vi "题目1.vi"() -> ()   [LabVIEW 2017]
panel:
  out "?":bool
  out "倒计时":string
  in  "停止":bool
  in  "开始计时":bool
  in  "定时时间选择":enum16{"90秒", "6秒", "10秒", "20秒"}(ring)
  # "倒 计 时 器"
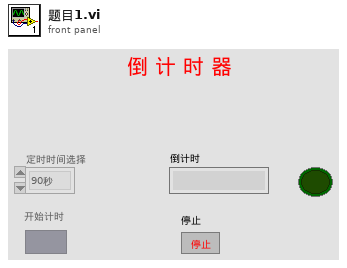
[diagram p1: front panel]
types:
  T1 = enum8{"Enabled", "Disabled", "Disabled and Grayed Out"}
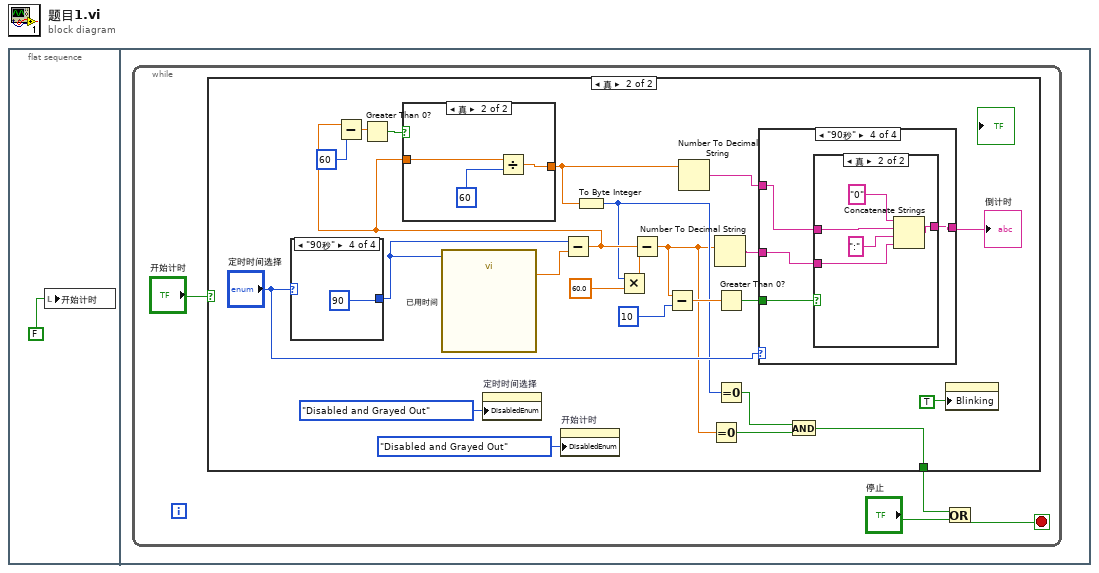
[diagram p0: block diagram]
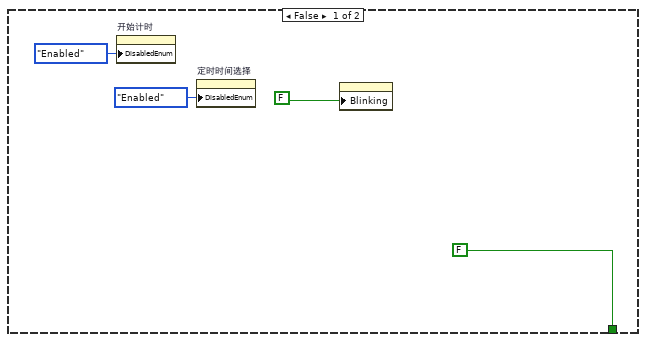
[diagram p2: hidden frame]
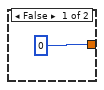
[diagram p3: hidden frame]
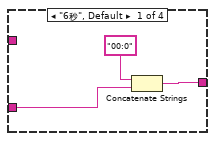
[diagram p4: hidden frame]
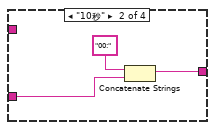
[diagram p5: hidden frame]
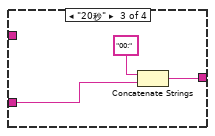
[diagram p6: hidden frame]
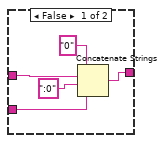
[diagram p7: hidden frame]
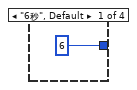
[diagram p8: hidden frame]
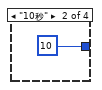
[diagram p9: hidden frame]
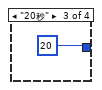
[diagram p10: hidden frame]
diagram:
  n1 = flat-sequence {
    frame #0 {
      n2 = local write "开始计时"(FALSE ("布尔")) -> ()
    }
    frame #1 {
      n3 = while {
        stop <- w2 stop-if-true
        n4 = case shown="真" "开始计时" {
          tunnel: [FALSE w12] -> w4
          frame False {
            n5 = property on="开始计时" class="Bool (严格)"("DisabledEnum"=T1."Enabled" ("禁用")) -> ()  [unwired: 2 in, 2 out]
            n6 = property on="定时时间选择" class="Enum (严格)"("DisabledEnum"=T1."Enabled" ("禁用")) -> ()  [unwired: 2 in, 2 out]
            n7 = property class="Bool (严格)"("Blinking"=FALSE ("闪烁")) -> ()  [unwired: 2 in, 2 out]
          }
          frame True {
            n8 = case shown="\"90秒\"" "定时时间选择" {
              tunnel: [6 10 20 90] -> w27
              frame "6秒", Default {
              }
              frame "10秒" {
              }
              frame "20秒" {
              }
              frame "90秒" {
              }
            }
            n9 = call "已用时间"("Time Target (s)"=w27) -> ("Elapsed Time (s)"=w25:dbl)  [unwired: 11 in, 7 out]
            n10 = property on="定时时间选择" class="Enum (严格)"("DisabledEnum"=T1."Disabled and Grayed Out" ("禁用")) -> ()  [unwired: 2 in, 2 out]
            n11 = property on="开始计时" class="Bool (严格)"("DisabledEnum"=T1."Disabled and Grayed Out" ("禁用")) -> ()  [unwired: 2 in, 2 out]
            n12 = Subtract(x=w27, y=w25) -> (x-y=w18:dbl)
            n13 = Subtract(x=w18, y=60) -> (x-y=w29:dbl)
            n14 = Greater Than 0?(x=w29) -> (x > 0?=w28:bool)
            n15 = case shown="真" w28 {
              tunnel: w18 -> [_ w37]
              tunnel: [0 w35] -> w22
              frame False {
              }
              frame True {
                n16 = Divide(x=w37, y=60) -> (x/y=w35:dbl)
              }
            }
            n17 = To Byte Integer(number=w22) -> (8bit integer=w14:i8)
            n18 = Multiply(x=w14, y=60.0) -> (x*y=w24:dbl)
            n19 = Subtract(x=w18, y=w24) -> (x-y=w11:dbl)
            n20 = Subtract(x=w11, y=10) -> (x-y=w20:dbl)
            n21 = Number To Decimal String(number=w22) -> (decimal integer string=w26:string)  [unwired: 1 in]
            n22 = Equal To 0?(x=w11) -> (x = 0?=w10:bool)
            n23 = Number To Decimal String(number=w11) -> (decimal integer string=w32:string)  [unwired: 1 in]
            n24 = Greater Than 0?(x=w20) -> (x > 0?=w19:bool)
            n25 = Equal To 0?(x=w14) -> (x = 0?=w13:bool)
            n26 = case shown="\"90秒\"" "定时时间选择" {
              tunnel: w32 -> [w39 w42 w45 w48]
              tunnel: [w38 w41 w44 w49] -> w31
              tunnel: w26 -> [_ _ _ w50]
              tunnel: w19 -> [_ _ _ w47]
              frame "6秒", Default {
                n27 = Concatenate Strings("00:0", w39) -> (w38:string)
              }
              frame "10秒" {
                n28 = Concatenate Strings("00:", w42) -> (w41:string)
              }
              frame "20秒" {
                n29 = Concatenate Strings("00:", w45) -> (w44:string)
              }
              frame "90秒" {
                n30 = case shown="真" w47 {
                  tunnel: w50 -> [w53 w58]
                  tunnel: [w51 w57] -> w49
                  tunnel: w48 -> [w52 w56]
                  frame False {
                    n31 = Concatenate Strings("0", w53, ":0", w52) -> (w51:string)
                  }
                  frame True {
                    n32 = Concatenate Strings("0", w58, ":", w56) -> (w57:string)
                  }
                }
              }
            }
            "倒计时" <- w31
            n33 = And(x=w13, y=w10) -> (x .and. y?=w12:bool)
            n34 = property class="Bool (严格)"("Blinking"=TRUE ("闪烁")) -> ()  [unwired: 2 in, 2 out]
          }
        }
        n35 = Or(x=w4, y="停止") -> (x .or. y?=w2:bool)
      }
    }
  }
